vi "BRig_Host__Loop_Producer__tcp_System__Data_getExpPrefix.vi"(0 "input_strCmd":string) -> (14 "output_expPrefix":string, 15 "output_I_expPrefix":bool)   [LabVIEW 2014]
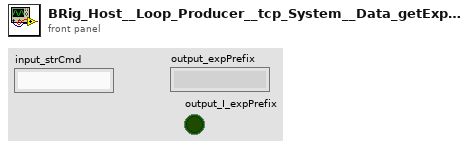
[diagram p1: front panel]
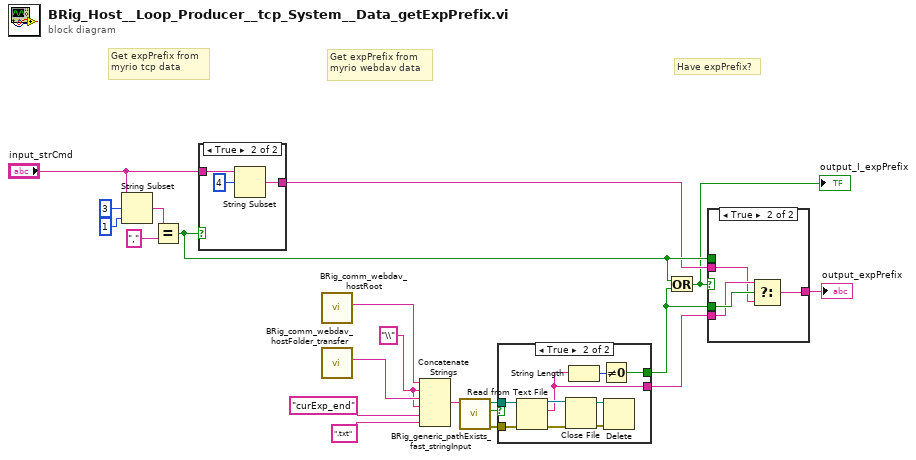
[diagram p0: block diagram]
diagram:
  w13 = "\\" ("string")
  # "Have expPrefix?"
  # "Get expPrefix from\nmyrio webdav data"
  # "Get expPrefix from\nmyrio tcp data"
  n1 = String Subset(string="input_strCmd", offset (0)=3, length (rest)=1 ("offset (0)")) -> (substring=w18:string)
  n2 = Equal?(x=w18, y=",") -> (x = y?=w6:bool)
  n3 = case shown="True" w6 {
    tunnel: "input_strCmd" -> [_ w23]
    tunnel: [_ w21] -> w4
    frame False {
    }
    frame True {
      n4 = String Subset(string=w23, offset (0)=4) -> (substring=w21:string)  [unwired: 1 in]
    }
  }
  n5 = call "BRig_comm_webdav_hostRoot.vi"() -> ("output_hostRoot"=w14:string)  [unwired: 11 in]
  n6 = call "BRig_comm_webdav_hostFolder_transfer.vi"() -> ("output_HostFolder"=w15:string)  [unwired: 11 in]
  n7 = Concatenate Strings(w14, w13, w15, w13, "curExp_end" ("intput_fileName"), ".txt" ("string")) -> (w10:string)
  n8 = call "BRig_generic_pathExists_fast_stringInput.vi"("input_filePath"=w10) -> ("output_error"=w7:errorcluster, "output_Iexist"=w9:bool, "output_filePath"=w8:path)  [unwired: 8 in]
  n9 = case shown="True" w9 {
    tunnel: w8 -> [_ w28]
    tunnel: w7 -> [_ w27]
    tunnel: [_ w25] -> w5
    tunnel: [_ w24] -> w3
    frame False {
    }
    frame True {
      n10 = Read from Text File(file (use dialog)=w28, error in=w27) -> (refnum out=w29:refnum<file>, text=w24:string, error out=w30:errorcluster)  [unwired: 2 in, 1 out]
      n11 = Close File(refnum=w29, error in=w30) -> (path=w31:path, error out=w32:errorcluster)
      n12 = String Length(string=w24) -> (length=w26:i32)
      n13 = Not Equal To 0?(x=w26) -> (x != 0?=w25:bool)
      n14 = Delete(path (use dialog)=w31, error in=w32) -> ()  [unwired: 3 in, 3 out]
    }
  }
  n15 = Or(x=w6, y=w5) -> (x .or. y?=w1:bool)
  "output_I_expPrefix" <- w1
  n16 = case shown="True" w1 {
    tunnel: w6 -> [_ _]
    tunnel: w5 -> [_ w36]
    tunnel: w4 -> [_ w34]
    tunnel: w3 -> [_ w35]
    tunnel: [_ w33] -> w2
    frame False {
    }
    frame True {
      n17 = Select(t=w35, s=w36, f=w34) -> (s? t:f=w33:string)
    }
  }
  "output_expPrefix" <- w2
